vi "isolation_test_replace_empty.vi"(10 "Isulation test 2":string, 11 "Isulation test 1":string) -> (2 "Isulation test 2":string, 3 "Isulation test 1":string)   [LabVIEW 2021]
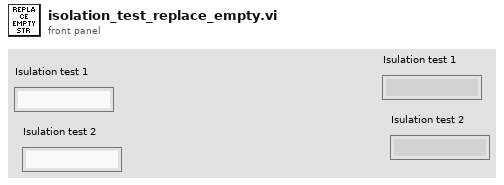
[diagram p1: front panel]
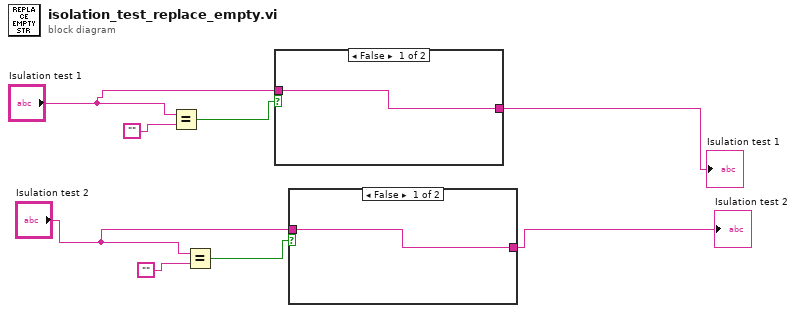
[diagram p0: block diagram]
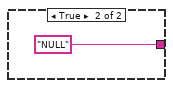
[diagram p2: hidden frame]
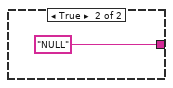
[diagram p3: hidden frame]
diagram:
  n1 = Equal?(x="Isulation test 1", y="") -> (x = y?=w7:bool)
  n2 = Equal?(x="Isulation test 2", y="") -> (x = y?=w4:bool)
  n3 = case shown="False" w7 {
    tunnel: [w9 "NULL"] -> w6
    tunnel: "Isulation test 1" -> [w9 _]
    frame False {
    }
    frame True {
    }
  }
  "Isulation test 1" <- w6
  n4 = case shown="False" w4 {
    tunnel: [w11 "NULL"] -> w1
    tunnel: "Isulation test 2" -> [w11 _]
    frame False {
    }
    frame True {
    }
  }
  "Isulation test 2" <- w1
